vi "Escape.vi"(11 "string":string) -> (3 "escaped string":string)   [LabVIEW 2019, in "JSON.lvlib"]
doc: "Escapes a JSON string:\n \\b = Backspace (0x08)\n \\f = Form feed (0x0C)\n \\n = New line (0x0A)\n \\r = Carriage return (0x0D)\n \\t = Tab (0x09)\n \\\" = Double quote (0x22)\n \\\\ = Backslash character (0x5C)\n\nCreated by: Ryan Pacini"
uses:
  JSON.lvlib
panel:
  out "characters escaped?":bool
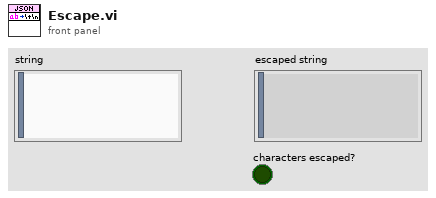
[diagram p1: front panel]
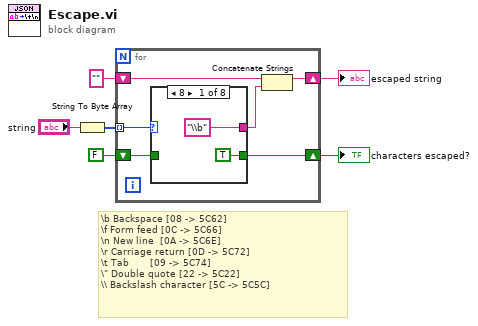
[diagram p0: block diagram]
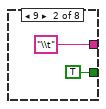
[diagram p2: hidden frame]
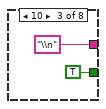
[diagram p3: hidden frame]
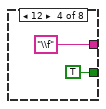
[diagram p4: hidden frame]
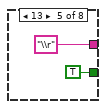
[diagram p5: hidden frame]
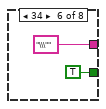
[diagram p6: hidden frame]
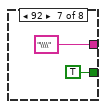
[diagram p7: hidden frame]
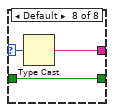
[diagram p8: hidden frame]
diagram:
  # "\\b Backspace [08 -> 5C62]\n\\f Form feed [0C -> 5C66]\n\\n New line  [0A -> 5C6E]\n\\r Carriage return [0D -> 5C72]\n\\t Tab       [09 -> 5C74]\n\\\" Double quote [22 -> 5C22]\n\\\\ Backslash character [5C -> 5C5C]"
  n1 = String To Byte Array(string="string") -> (unsigned byte array=w3:u8[])
  n2 = for {
    shift-right: [w10] -> w5
    shift-left: "" -> [w11]
    tunnel: w3 -> [w12] mode=indexing
    shift-right: [w8] -> w2
    shift-left: FALSE -> [w7]
    n3 = case shown="8" w12 {
      selector: w12 -> [_ _ _ _ _ _ _ w29]
      tunnel: ["\\b" "\\t" "\\n" "\\f" "\\r" "\\\"" "\\\\" w28] -> w9
      tunnel: [TRUE TRUE TRUE TRUE TRUE TRUE TRUE w27] -> w8
      tunnel: w7 -> [_ _ _ _ _ _ _ w27]
      frame 8 {
      }
      frame 9 {
      }
      frame 10 {
      }
      frame 12 {
      }
      frame 13 {
      }
      frame 34 {
      }
      frame 92 {
      }
      frame Default {
        n4 = Type Cast(x=w29) -> (*(type *) &x=w28:string)  [unwired: 1 in]
      }
    }
    n5 = Concatenate Strings(w11, w9) -> (w10:string)
  }
  "escaped string" <- w5
  "characters escaped?" <- w2
